vi "Get Fruit Color.vi"(2 "Fruit in":refnum<class "Fruit.lvclass">) -> (7 "FruitColor":u32(colorbox)=16728794)   [LabVIEW 2021, in "Fruit.lvclass"]
uses:
  Fruit.lvclass
  Fruit.lvclass/Fruit.ctl
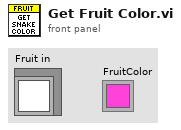
[diagram p1: front panel]
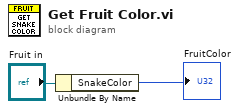
[diagram p0: block diagram]
diagram:
  n1 = Unbundle By Name("Fruit in") -> ("SnakeColor"=→"FruitColor":u32)
